vi "Cryo-Con Set Control.vi"(8 "error in (no error)":errorcluster, 10 "Set T":T1=enum."0.25W", 11 "VISA Resource Name":refnum<visa-resource-name>) -> (0 "error out":errorcluster, 3 "VISA Resource Name Out":refnum<visa-resource-name>)   [LabVIEW 2015]
uses:
  Cryo-con Heater Ranges.ctl
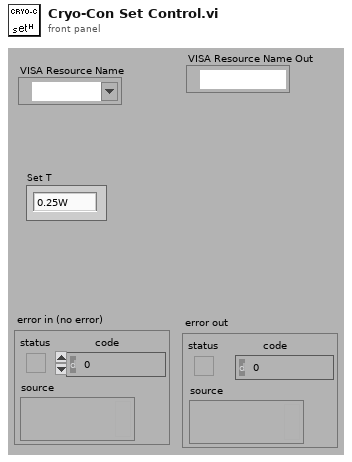
[diagram p1: front panel]
types:
  T1 = typedef "Cryo-con Heater Ranges.ctl" = enum16{"25W", "2.5W", "0.25W"}
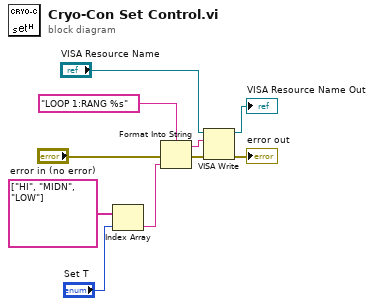
[diagram p0: block diagram]
diagram:
  n1 = Index Array(array=string[] ["HI", "MIDN", "LOW"] ("string array"), index="Set T") -> (element=w1:string)
  n2 = Format Into String(format string="LOOP 1:RANG %s", error in="error in (no error)", w1) -> (resulting string=w6:string, error out=w8:errorcluster)  [unwired: 1 in]
  n3 = VISA Write(VISA resource name="VISA Resource Name", write buffer=w6, error in (no error)=w8) -> (VISA resource name out=→"VISA Resource Name Out":refnum<visa-resource-name>, error out=→"error out":errorcluster)  [unwired: 1 out]
